vi "Insert Coin.vi"(0 "reference in":refnum<class "No Coin State.lvclass">, 5 "error in (no error)":errorcluster) -> (14 "reference out":refnum<class "No Coin State.lvclass">, 19 "error out":errorcluster)   [LabVIEW 2013, in "No Coin State.lvclass"]
uses:
  No Coin State.lvclass
  Gum Machine_class/Gum Machine.lvclass
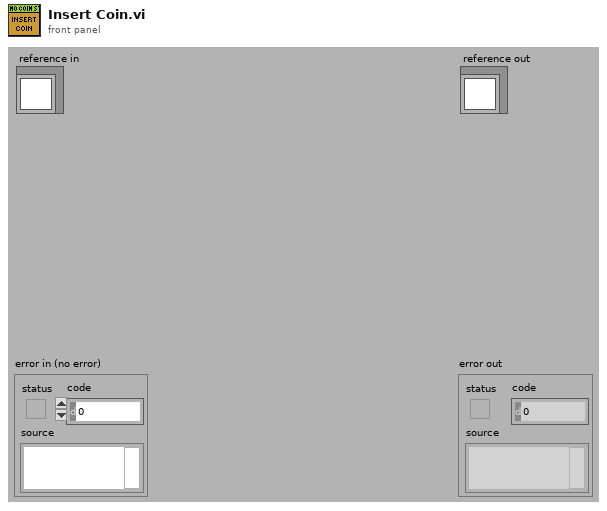
[diagram p1: front panel]
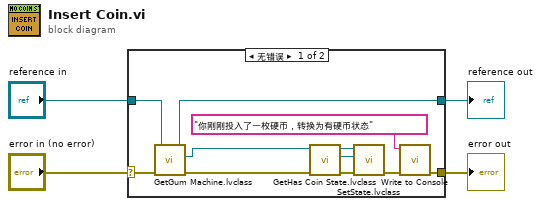
[diagram p0: block diagram]
diagram:
  n1 = case shown="无错误" "error in (no error)" {
    selector: "error in (no error)" -> [w11 w17]
    tunnel: [w8 w17] -> w3
    tunnel: [w7 w16] -> w1
    tunnel: "reference in" -> [w14 w16]
    frame No Error {
      n2 = call-dynamic "GetGum Machine.lvclass.vi"("error in (no error)"=w11, "reference in"=w14) -> ("error out"=w6:errorcluster, "Gum Machine.lvclass"=w5:refnum<class "Gum Machine.lvclass">, "reference out"=w7:refnum<class "No Coin State.lvclass">)  [unwired: 7 in]
      n3 = call-dynamic "GetHas Coin State.lvclass.vi"("error in (no error)"=w6, "reference in"=w5) -> ("error out"=w10:errorcluster, "Has Coin State.lvclass"=w13:refnum<class "Has Coin State.lvclass">, "reference out"=w12:refnum<class "Gum Machine.lvclass">)  [unwired: 7 in]
      n4 = call-dynamic "SetState.lvclass.vi"("error in (no error)"=w10, "State.lvclass"=w13, "reference in"=w12) -> ("error out"=w9:errorcluster)  [unwired: 7 in, 1 out]
      n5 = call "Write to Console.vi"("error in (no error)"=w9, "Input"="你刚刚投入了一枚硬币，转换为有硬币状态") -> ("error out"=w8:errorcluster)  [unwired: 9 in]
    }
    frame Error {
    }
  }
  "error out" <- w3
  "reference out" <- w1
